vi "Tweet with Image.vi"(9 "Picture File (PNG, JPG, GIF)":path, 10 "Tweet":string="@RockcrusadersO") -> (0 "error out":errorcluster)   [LabVIEW 2020, in "Twitter.lvclass"]
uses:
  Twitter.lvclass
  <vilib>/LVH/i3 OAuth/Controls/Credentials.ctl
  <vilib>/LVH/i3 Twitter/SubVIs/Twitter Open - Desktop.vi
  <vilib>/LVH/i3 Twitter/Tweets with Media/Post Media Tweet - From File.vi
  <vilib>/LVH/i3 Twitter/i3-twitter.lvlib
  <vilib>/LVH/i3 OAuth/i3-oauth.lvlib
panel:
  out "Access Credentials (out)":T1
  in  "Consumer Key":string="Kn7UN5TS1O9UciZbi7tq5bSir"
  in  "Consumer Secret":string="tGV6hXiREzXobIISuOnVjCSuF8uaWDGQ2wft4uNlem4sOlMHcz"
  in  "Access Credentials (in)":T1={"Token"="188800942-G5ZRgZ7lorIJfOdNhAsnVTpF2nfCG000TN6KQ8WY", "Secret"="hbl24ankOLK3ZM6Qa3HbU3BZoSbWz0iciJ1tzBQGcj6SS"}
  in  "error in":errorcluster
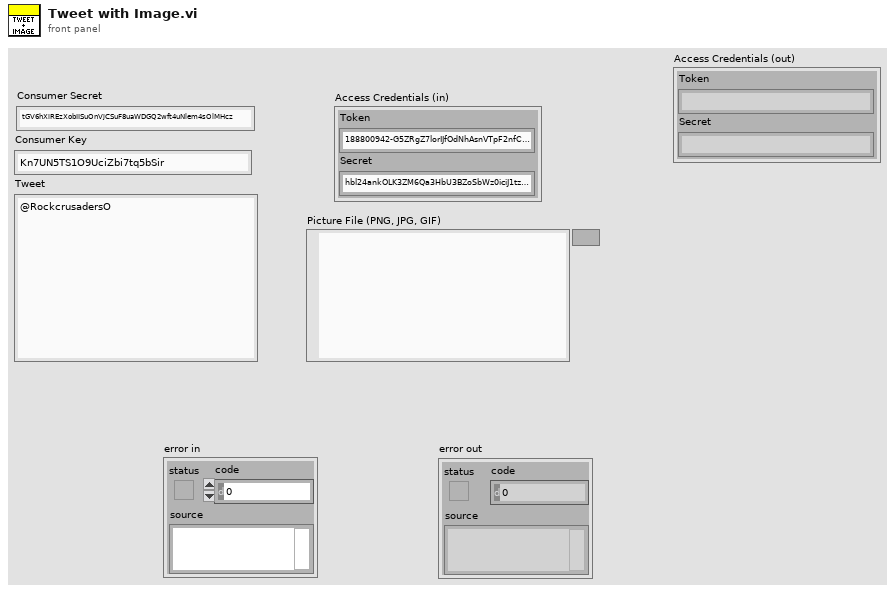
[diagram p1: front panel]
types:
  T1 = typedef "i3-oauth.lvlib/Credentials.ctl" = cluster{"Token":string, "Secret":string}
  T2 = typedef "i3-twitter.lvlib/Twitter Handle.ctl" = cluster{"OAuth Credentials":T3, "since ID":string, "max ID":string, "Screen Name":string}
  T3 = typedef "i3-oauth.lvlib/OAuth Handle.ctl" = cluster{"Signature Method":T4, "Version":string, "Client":T1, "Access":T1}
  T4 = typedef "i3-oauth.lvlib/Signature Method.ctl" = enum16{"HMAC-MD5", "HMAC-SHA1", "HMAC-SHA224", "HMAC-SHA256", "HMAC-SHA384", "HMAC-SHA512"}
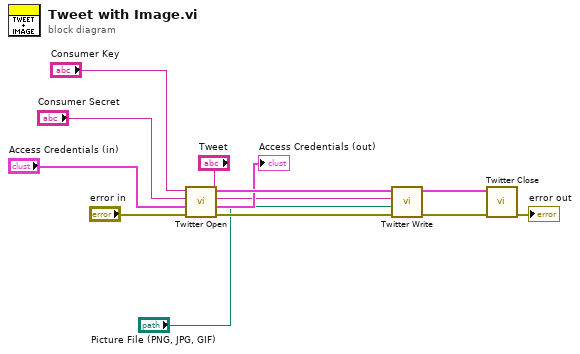
[diagram p0: block diagram]
diagram:
  n1 = call-poly <vilib>:"Twitter Open.vi"("error in"="error in", "Access Credentials (in)"="Access Credentials (in)", "Consumer Secret"="Consumer Secret", "Consumer Key"="Consumer Key") -> ("error out"=w5:errorcluster, "Access Credentials (out)"=→"Access Credentials (out)":T1, "Twitter Handle Out"=w11:T2)  [unwired: 5 in]
  n2 = call-poly <vilib>:"Twitter Write.vi"("error in"=w5, "Picture File (PNG, JPG, GIF)"="Picture File (PNG, JPG, GIF)", "Tweet"="Tweet", "Twitter Handle In"=w11) -> ("error out"=w4:errorcluster, "Twitter Handle Out"=w12:T2)  [unwired: 6 in]
  n3 = call <vilib>:"Twitter Close.vi"("error in"=w4, "Twitter Handle In"=w12) -> ("error out"=→"error out":errorcluster)  [unwired: 9 in]
